vi "Readwindowpropfile.vi"(11 "configuration file path":path) -> (0 "PanelOrigin":cluster{"panelx":i16, "panely":i16}, 1 "MinimumSize":cluster{"Horizontal":i16, "Vertical":i16}, 2 "PanelBounds":T1, 3 "resizable":bool, 4 "AllFound":bool)   [LabVIEW 2019]
uses:
  <vilib>/Utility/config.llb/Read Key (Boolean).vi
  <vilib>/Utility/config.llb/Read Key (I32).vi
  <vilib>/Utility/config.llb/NI_LVConfig.lvlib
panel:
  out "Message":string
  out "Error":bool
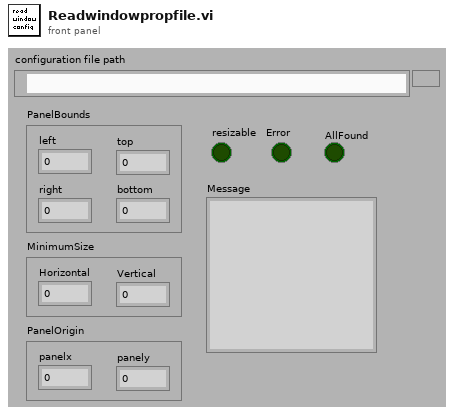
[diagram p1: front panel]
types:
  T1 = cluster{"left":i16, "top":i16, "right":i16, "bottom":i16}
  T2 = typedef "NI_LVConfig.lvlib/Config Data RefNum.ctl" = refnum<k1>
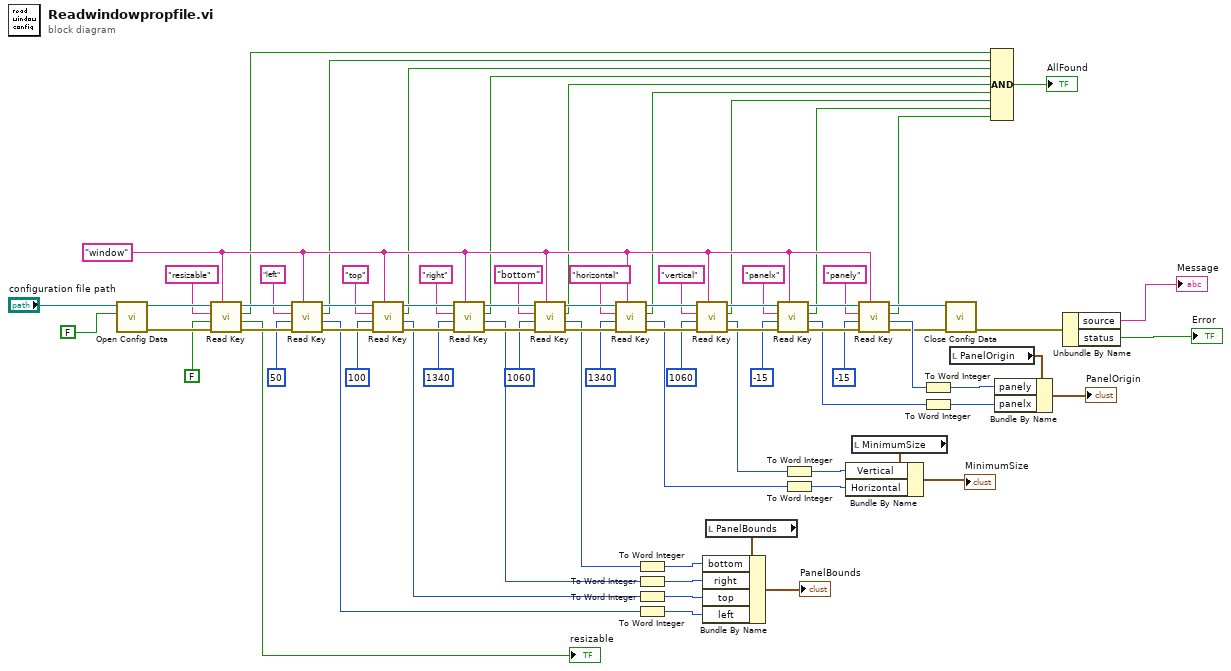
[diagram p0: block diagram]
diagram:
  w58 = "window" ("section")
  n1 = call <vilib>:"Open Config Data.vi"("create file if necessary (T)"=FALSE, "configuration file path"="configuration file path") -> ("error out"=w76:errorcluster, "refnum"=w77:T2)  [unwired: 7 in, 1 out]
  n2 = call-poly <vilib>:"Read Key.vi"("section"=w58, "error in (no error)"=w76, "default value"=FALSE, "key"="resizable", "refnum"=w77) -> ("error out"=w73:errorcluster, "value"=→"resizable":bool, "found?"=w10:bool, "refnum out"=w74:T2)  [unwired: 3 in]
  n3 = call-poly <vilib>:"Read Key.vi"("section"=w58, "error in (no error)"=w73, "default value"=50, "key"="left", "refnum"=w74) -> ("error out"=w71:errorcluster, "value"=w47:i32, "found?"=w9:bool, "refnum out"=w72:T2)  [unwired: 3 in]
  n4 = call-poly <vilib>:"Read Key.vi"("section"=w58, "error in (no error)"=w71, "default value"=100, "key"="top", "refnum"=w72) -> ("error out"=w61:errorcluster, "value"=w46:i32, "found?"=w8:bool, "refnum out"=w62:T2)  [unwired: 3 in]
  n5 = call-poly <vilib>:"Read Key.vi"("section"=w58, "error in (no error)"=w61, "default value"=1340, "key"="right", "refnum"=w62) -> ("error out"=w68:errorcluster, "value"=w45:i32, "found?"=w7:bool, "refnum out"=w67:T2)  [unwired: 3 in]
  n6 = call-poly <vilib>:"Read Key.vi"("section"=w58, "error in (no error)"=w68, "default value"=1060, "key"="bottom", "refnum"=w67) -> ("error out"=w70:errorcluster, "value"=w44:i32, "found?"=w6:bool, "refnum out"=w69:T2)  [unwired: 3 in]
  n7 = call-poly <vilib>:"Read Key.vi"("section"=w58, "error in (no error)"=w70, "default value"=1340, "key"="horizontal", "refnum"=w69) -> ("error out"=w59:errorcluster, "value"=w37:i32, "found?"=w5:bool, "refnum out"=w60:T2)  [unwired: 3 in]
  n8 = To Word Integer(number=w44) -> (16bit integer=w42:i16)
  n9 = To Word Integer(number=w45) -> (16bit integer=w41:i16)
  n10 = To Word Integer(number=w46) -> (16bit integer=w40:i16)
  n11 = To Word Integer(number=w47) -> (16bit integer=w39:i16)
  n12 = call-poly <vilib>:"Read Key.vi"("section"=w58, "error in (no error)"=w59, "default value"=1060, "key"="vertical", "refnum"=w60) -> ("error out"=w65:errorcluster, "value"=w36:i32, "found?"=w4:bool, "refnum out"=w66:T2)  [unwired: 3 in]
  n13 = local read "PanelBounds"() -> (w43:T1)
  n14 = Bundle By Name(cluster=w43, "bottom"=w42, "right"=w41, "top"=w40, "left"=w39) -> (→"PanelBounds":T1)
  n15 = call-poly <vilib>:"Read Key.vi"("section"=w58, "error in (no error)"=w65, "default value"=-15, "key"="panelx", "refnum"=w66) -> ("error out"=w63:errorcluster, "value"=w35:i32, "found?"=w3:bool, "refnum out"=w64:T2)  [unwired: 3 in]
  n16 = To Word Integer(number=w36) -> (16bit integer=w30:i16)
  n17 = To Word Integer(number=w37) -> (16bit integer=w31:i16)
  n18 = local read "MinimumSize"() -> (w33:cluster{"Horizontal":i16, "Vertical":i16})
  n19 = Bundle By Name(cluster=w33, "Vertical"=w30, "Horizontal"=w31) -> (→"MinimumSize":cluster{"Horizontal":i16, "Vertical":i16})
  n20 = call-poly <vilib>:"Read Key.vi"("section"=w58, "error in (no error)"=w63, "default value"=-15, "key"="panely", "refnum"=w64) -> ("error out"=w23:errorcluster, "value"=w34:i32, "found?"=w2:bool, "refnum out"=w22:T2)  [unwired: 3 in]
  n21 = To Word Integer(number=w34) -> (16bit integer=w28:i16)
  n22 = To Word Integer(number=w35) -> (16bit integer=w27:i16)
  n23 = call <vilib>:"Close Config Data.vi"("error in (no error)"=w23, "refnum"=w22) -> ("error out"=w21:errorcluster)  [unwired: 8 in, 1 out]
  n24 = local read "PanelOrigin"() -> (w29:cluster{"panelx":i16, "panely":i16})
  n25 = Compound Arithmetic op=AND(w10, w9, w8, w7, w6, w5, w4, w3, w2) -> (→"AllFound":bool)
  n26 = Bundle By Name(cluster=w29, "panely"=w28, "panelx"=w27) -> (→"PanelOrigin":cluster{"panelx":i16, "panely":i16})
  n27 = Unbundle By Name(w21) -> ("source"=→"Message":string, "status"=→"Error":bool)
